vi "PCO_GetDelayExposureTimeTable.vi"(8 "error in (no error)":errorcluster {"code" format="%x"}, 11 "ph":u64) -> (0 "error out":errorcluster {"code" format="%x"}, 1 "dwDelay":u32[](array[numeric]), 2 "ErrorMessage":i32 format="%x", 3 "ph out":u64, 4 "wTimeBaseDelay":u16(ring) items=["ns", "us", "ms"], 5 "dwExposure":u32[](array[numeric]), 7 "wTimeBaseExposure":u16(ring) items=["ns", "us", "ms"])   [LabVIEW 2019, in "SDK.lvlib" / "TimingControl.lvlib"]
doc: "<b>Description:</b>\nThis function returns the current setting of the delay and exposure time table values and the associated time base values. Maximum size of each array is 16 DWORD entries. Returned values are only valid if the last timing command was PCO_SetDelayExposureTimeTable.\nSee PCO_SetDelayExposureTimeTable for a more detailed description of the delay / exposure time table usage.\n\n<b>Supported camera type:</b>\nAll cameras\n\n<b>Descriptor dependency:</b>\nwTimeTableDESC"
uses:
  TimingControl.lvlib
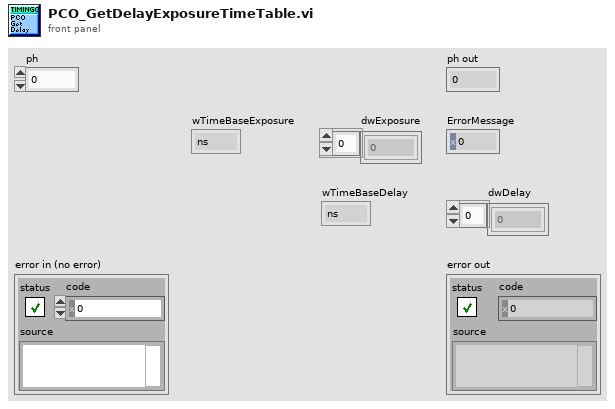
[diagram p1: front panel]
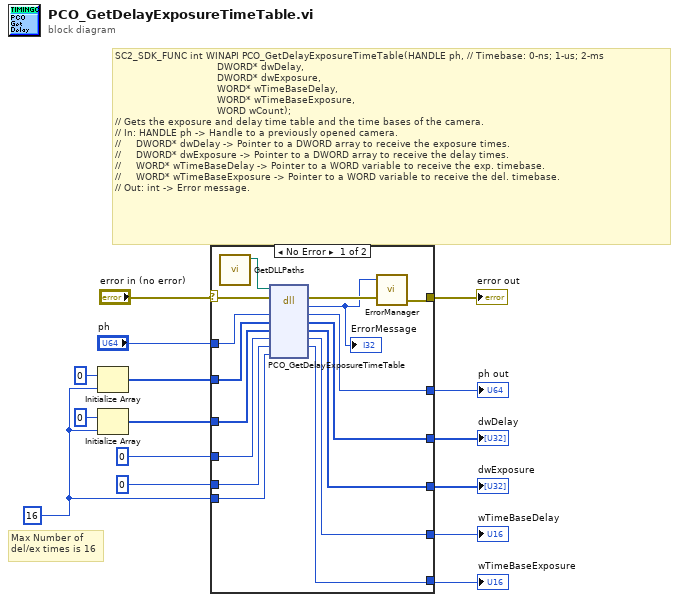
[diagram p0: block diagram]
diagram:
  w12 = u16 16 ("wCount")
  # "Max Number of \ndel/ex times is 16"
  # "SC2_SDK_FUNC int WINAPI PCO_GetDelayExposureTimeTable(HANDLE ph, // Timebase: 0-ns; 1-us; 2-ms \n                                  DWORD* dwDelay,\n                                  DWORD* dwExposure,\n                                  WORD* wTimeBaseDelay,\n                                  WORD* wTimeBaseExposure,\n                                  WORD wCount);\n// Gets the exposure and delay time table and the time bases of the camera.\n// In: HANDLE ph -> Handle to a previously opened camera.\n//     DWORD* dwDelay -> Pointer to a DWORD array to receive the exposure times.\n//     DWORD* dwExposure -> Pointer to a DWORD array to receive the delay times.\n//     WORD* wTimeBaseDelay -> Pointer to a WORD variable to receive the exp. timebase.\n//     WORD* wTimeBaseExposure -> Pointer to a WORD variable to receive the del. timebase.\n// Out: int -> Error message."
  n1 = Initialize Array(u32 0 ("element"), w12) -> (w13:u32[])
  n2 = Initialize Array(u32 0 ("element"), w12) -> (w9:u32[])
  n3 = case shown="No Error" "error in (no error)" {
    selector: "error in (no error)" -> [w20 w36]
    tunnel: "ph" -> [w31 w37]
    tunnel: [w30 w37] -> w14
    tunnel: w13 -> [w29 w35]
    tunnel: w12 -> [w28 _]
    tunnel: [w27 w35] -> w10
    tunnel: w9 -> [w26 w34]
    tunnel: [w25 w34] -> w7
    tunnel: u16 0 ("wTimeBaseDelay") -> [w24 w33]
    tunnel: [w23 w33] -> w5
    tunnel: u16 0 ("wTimeBaseExposure") -> [w22 w32]
    tunnel: [w21 w32] -> w3
    tunnel: [w18 w36] -> w2
    frame No Error {
      n4 = call "GetDLLPaths.vi"() -> ("SC2_Cam_Path"=w16:path)  [unwired: 9 in, 2 out]
      n5 = dll-call lib="?" fn="PCO_GetDelayExposureTimeTable"(path in=w16, error in=w20, "ph"=w31, "dwDelay"=w29, "dwExposure"=w26, "wTimeBaseDelay"=w24, "wTimeBaseExposure"=w22, "wCount"=w28) -> (error out=w19:errorcluster, "return type"=w17:i32, "ph"=w30:u64, "dwDelay"=w27:u32[], "dwExposure"=w25:u32[], "wTimeBaseDelay"=w23:u16, "wTimeBaseExposure"=w21:u16)  [unwired: 2 in, 1 out]
      "ErrorMessage" <- w17
      n6 = call "ErrorManager.vi"("error in (no error)"=w19, "error code"=w17) -> ("error out"=w18:errorcluster)  [unwired: 3 in]
    }
    frame Error {
    }
  }
  "ph out" <- w14
  "dwDelay" <- w10
  "dwExposure" <- w7
  "wTimeBaseDelay" <- w5
  "wTimeBaseExposure" <- w3
  "error out" <- w2
